vi "pannel-list-to-broadcaststring.vi"(11 "sce-pannel-list":T1(array[cluster])) -> (3 "sce-pannel-list-cmd":string)   [LabVIEW 2019]
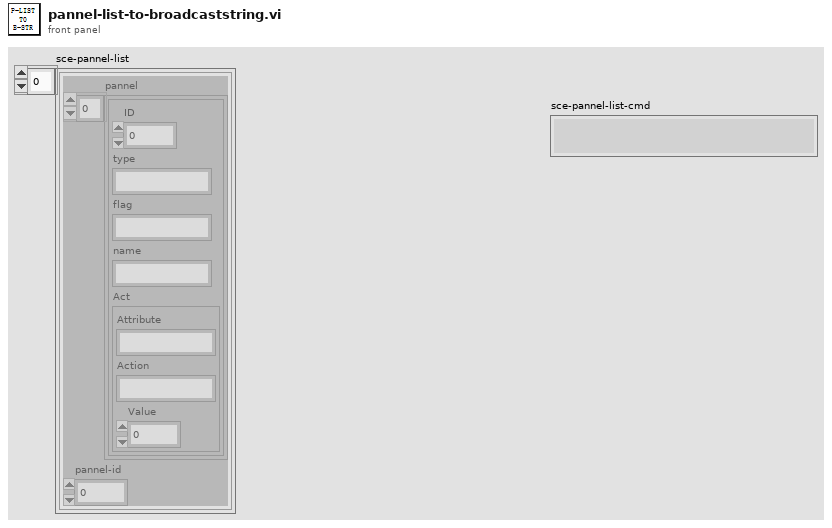
[diagram p1: front panel]
types:
  T1 = cluster{"pannel":cluster{"ID":u8, "type":string, "flag":string, "name":string, "Act":cluster{"Attribute":string, "Action":string, "Value":dbl}}[], "pannel-id":dbl}[]
  T2 = cluster{"ID":u8, "type":string, "flag":string, "name":string, "Act":cluster{"Attribute":string, "Action":string, "Value":dbl}}[]
  T3 = cluster{"pannel":cluster{"ID":u8, "type":string, "flag":string, "name":string, "Act":cluster{"Attribute":string, "Action":string, "Value":dbl}}[], "pannel-id":dbl}
  T4 = cluster{"ID":u8, "type":string, "flag":string, "name":string, "Act":cluster{"Attribute":string, "Action":string, "Value":dbl}}
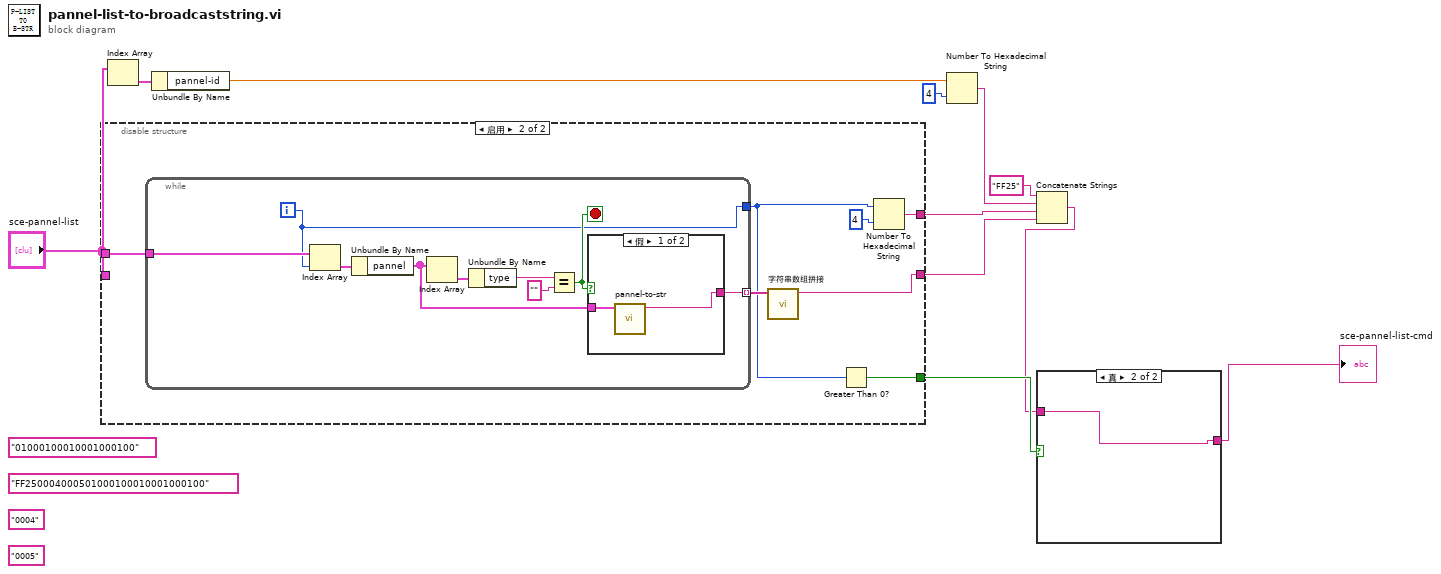
[diagram p0: block diagram]
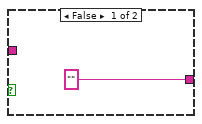
[diagram p2: hidden frame]
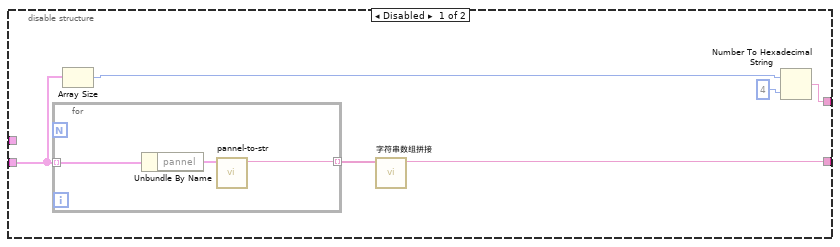
[diagram p3: hidden frame]
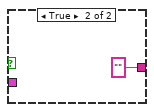
[diagram p4: hidden frame]
diagram:
  (unwired) "0005"
  (unwired) "01000100010001000100"
  (unwired) "0004"
  (unwired) "FF250004000501000100010001000100"
  n1 = disable-structure shown="启用" {
    disable-tunnel: [w16 w25] -> w9
    disable-tunnel: [w13 w23] -> w5
    disable-tunnel: "sce-pannel-list" -> [w12 _]
    disable-tunnel: "sce-pannel-list" -> [_ w27]
    disable-tunnel: [_ w21] -> w3
    frame Disabled {
      n2 = for {
        tunnel: w12 -> [w20] mode=indexing
        tunnel: [w18] -> w17 mode=indexing
        n3 = Unbundle By Name(w20) -> ("pannel"=w19:T2)
        n4 = call "pannel-to-str.vi"("pannel"=w19) -> ("字符串"=w18:string)  [unwired: 10 in]
      }
      n5 = Array Size(array=w12) -> (size(s)=w15:i32)
      n6 = call "字符串数组拼接.vi"("数组"=w17) -> ("字符串"=w16:string)  [unwired: 10 in]
      n7 = Number To Hexadecimal String(1:i16 4 ("宽度(-)"), 2:w15) -> (0:w13:string)
    }
    frame Enabled {
      n8 = while {
        tunnel: w27 -> [w36]
        tunnel: [w29] -> w26 mode=indexing
        tunnel: [w28] -> w22
        i -> [w28]
        stop <- w31 stop-if-true
        n9 = Index Array(array=w36, index=w28) -> (element=w35:T3)
        n10 = Unbundle By Name(w35) -> ("pannel"=w30:T2)
        n11 = Index Array(array=w30) -> (element=w34:T4)  [unwired: 1 in]
        n12 = Unbundle By Name(w34) -> ("type"=w33:string)
        n13 = Equal?(x=w33, y="") -> (x = y?=w31:bool)
        n14 = case shown="假" w31 {
          tunnel: w30 -> [w38 _]
          tunnel: [w37 "" ("字符串")] -> w29
          frame False {
            n15 = call "pannel-to-str.vi"("pannel"=w38) -> ("字符串"=w37:string)  [unwired: 10 in]
          }
          frame True {
          }
        }
      }
      n16 = call "字符串数组拼接.vi"("数组"=w26) -> ("字符串"=w25:string)  [unwired: 10 in]
      n17 = Greater Than 0?(x=w22) -> (x > 0?=w21:bool)
      n18 = Number To Hexadecimal String(1:i16 4 ("宽度(-)"), 2:w22) -> (0:w23:string)
    }
  }
  n19 = Index Array(array="sce-pannel-list") -> (element=w11:T3)  [unwired: 1 in]
  n20 = Unbundle By Name(w11) -> ("pannel-id"=w8:dbl)
  n21 = Number To Hexadecimal String(1:i16 4 ("宽度(-)"), 2:w8) -> (0:w6:string)
  n22 = Concatenate Strings("FF25", w6, w5, w9) -> (w2:string)
  n23 = case shown="真" w3 {
    tunnel: ["" w41] -> w1
    tunnel: w2 -> [_ w41]
    frame False {
    }
    frame True {
    }
  }
  "sce-pannel-list-cmd" <- w1
